vi "Test Cloneable API.vi"() -> ()   [LabVIEW 2024]
doc: "Cloneable API Tester."
uses:
  <vilib>/Utility/error.llb/DialogType.ctl
  <vilib>/JKI/JKI Simple Localization/Private/RegisterVIJKI_Simple_Localization.vi
  Cloneable.lvlib
  <vilib>/JKI/JKI Simple Localization/API/JKI Simple LocalizationJKI_Simple_Localization.lvlib
panel:
  out "last error":errorcluster
  in  "Show Diagram on Init":bool
  in  "wait for reply":bool=TRUE
  in  "Run as Singleton?":bool
  in  "Show Block Diagram":bool
  in  "Refresh Modules":bool
  in  "X":dbl=1.0
  out "Reply Payload":dbl
  out "Active Modules":string[](array[string])
  in  "Stop Module":bool
  in  "Select Module":i32(ring)=-1 caption="Select Module\nTo send Request to" items=["All"=-1, "1"=1, "2"=2, "3"=3, "4"=4, "5"=5, "6"=6, "7"=7, "8"=8, "9"=9, "10"=10]
  in  "Run New Module":bool
  out "Do Something Count":i32
  in  "Test Do Something Else and Wait for Reply":bool
  in  "Hide Module Panel":bool
  in  "Show Module Panel":bool caption="Show Panel"
  in  "Test Do Something Else":bool
  in  "Test Do Something":bool
  out "Status":string
  # "This VI tests the API for the Module."
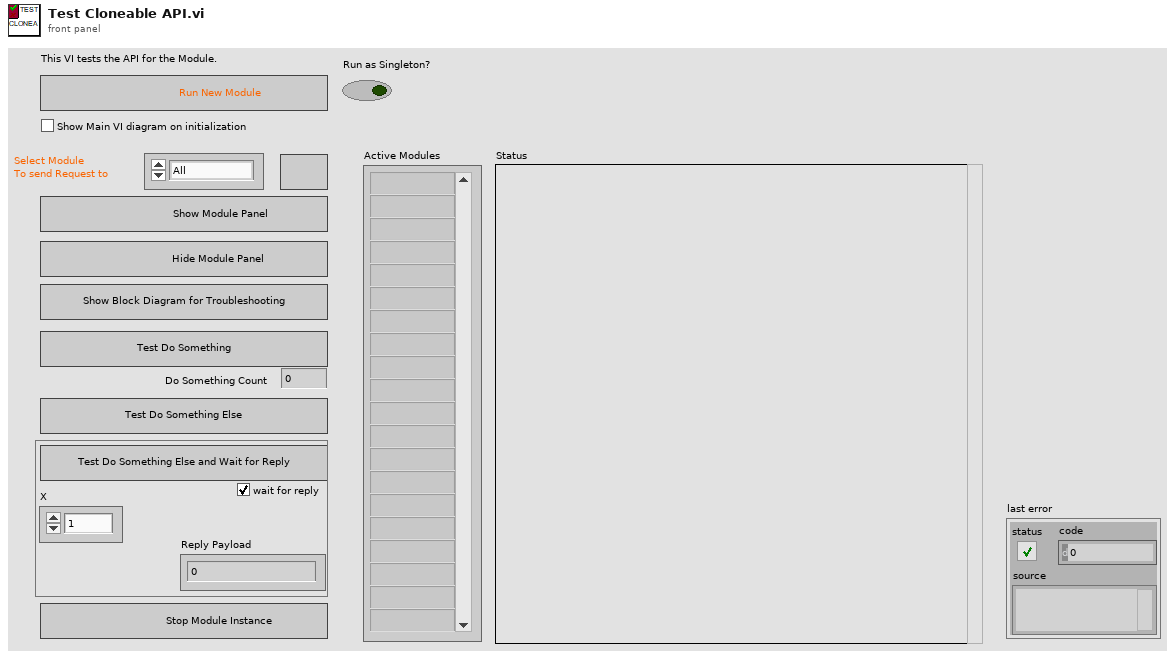
[diagram p1: front panel]
types:
  T1 = typedef "Cloneable.lvlib/Broadcast Events--cluster.ctl" = cluster{"Module Did Init":refnum<user-event>, "Status Updated":refnum<user-event>, "Error Reported":refnum<user-event>, "Did Something":refnum<user-event>, "Module Did Stop":refnum<user-event>, "Update Module Execution Status":refnum<user-event>}
  T2 = typedef "DialogType.ctl" = u16
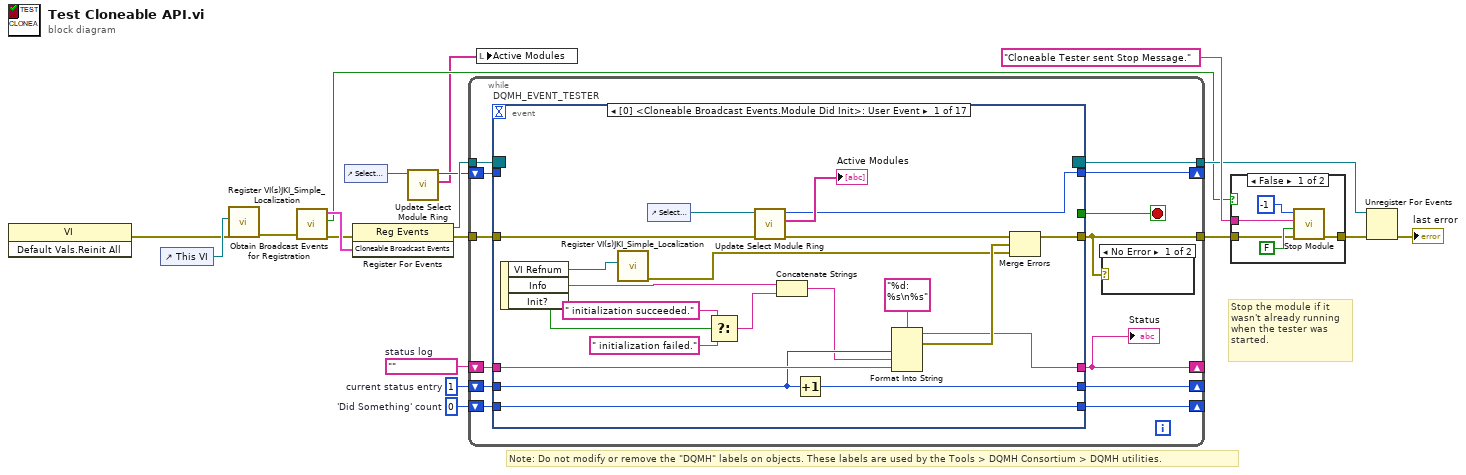
[diagram p0: block diagram]
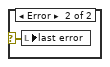
[diagram p3: hidden frame]
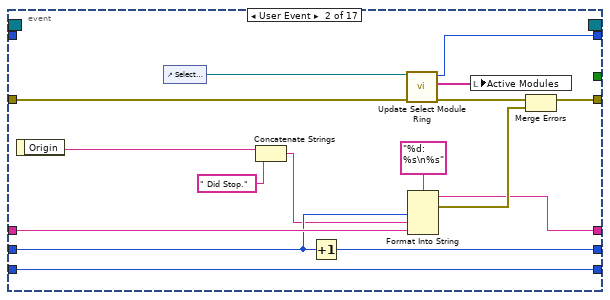
[diagram p4: hidden frame]
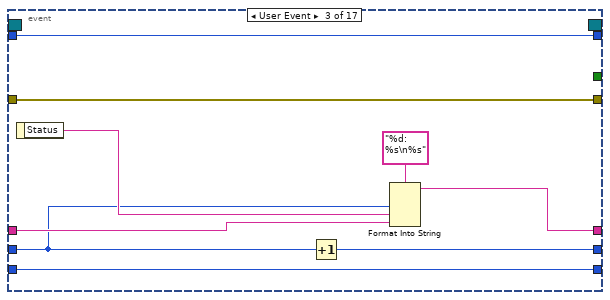
[diagram p5: hidden frame]
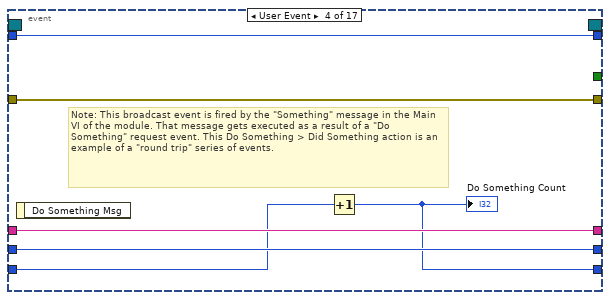
[diagram p6: hidden frame]
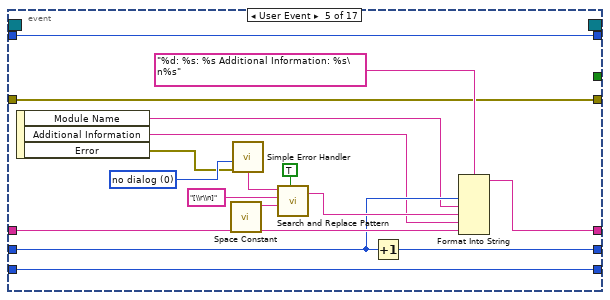
[diagram p7: hidden frame]
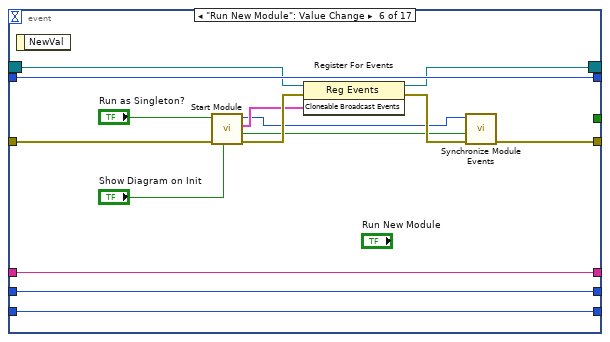
[diagram p8: hidden frame]
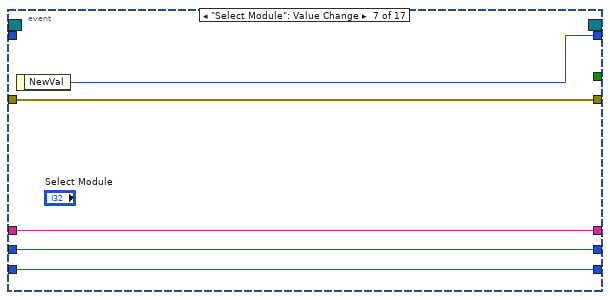
[diagram p9: hidden frame]
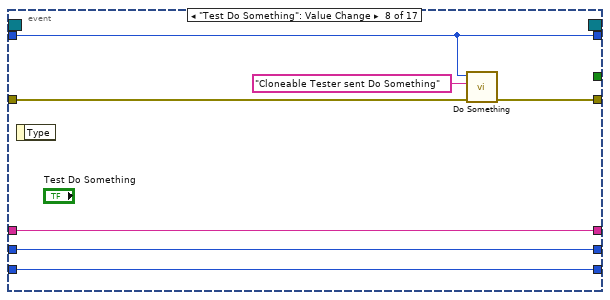
[diagram p10: hidden frame]
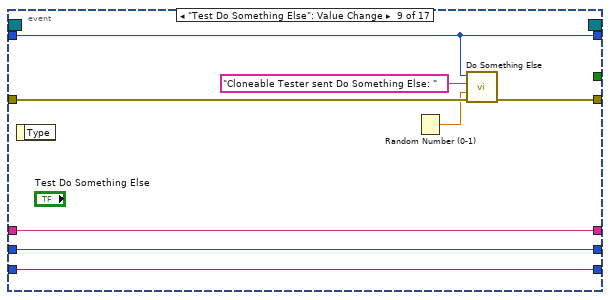
[diagram p11: hidden frame]
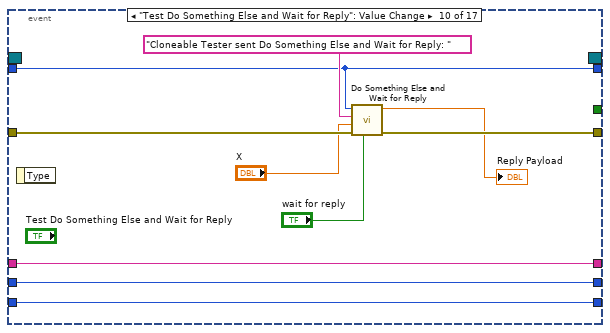
[diagram p12: hidden frame]
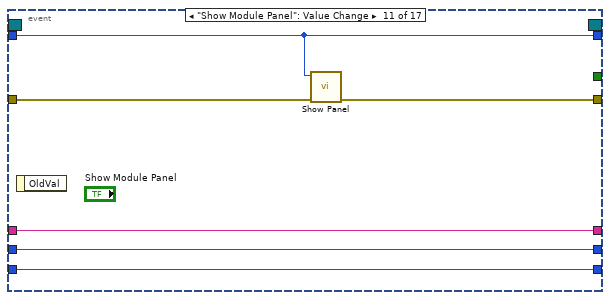
[diagram p13: hidden frame]
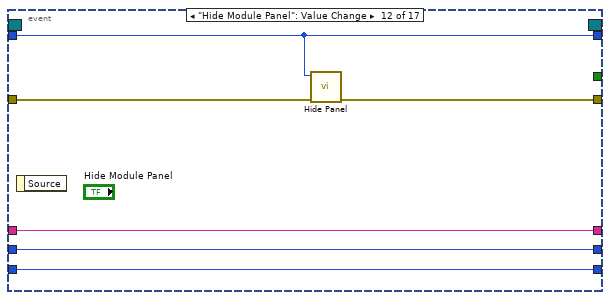
[diagram p14: hidden frame]
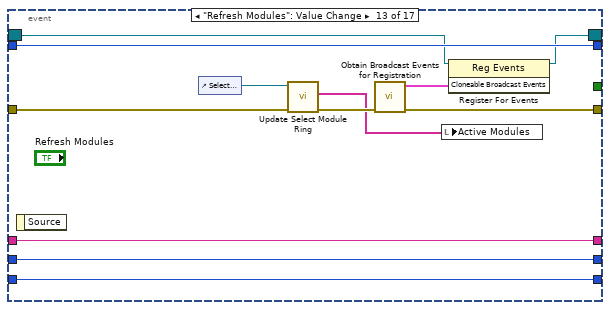
[diagram p15: hidden frame]
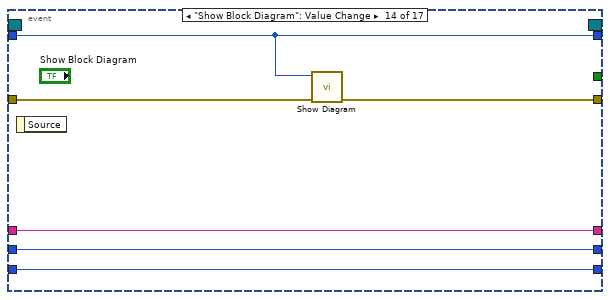
[diagram p16: hidden frame]
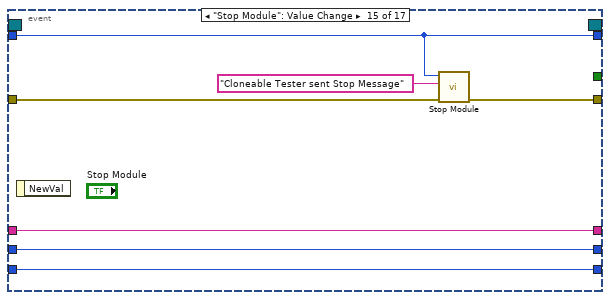
[diagram p17: hidden frame]
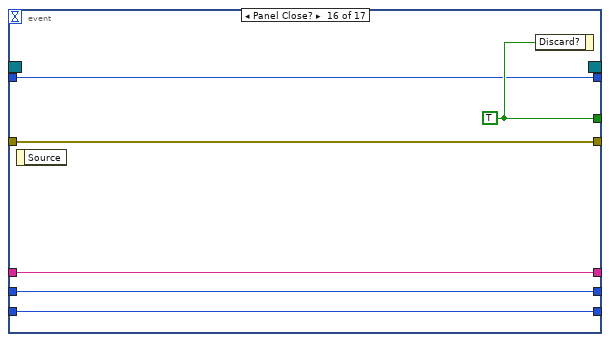
[diagram p18: hidden frame]
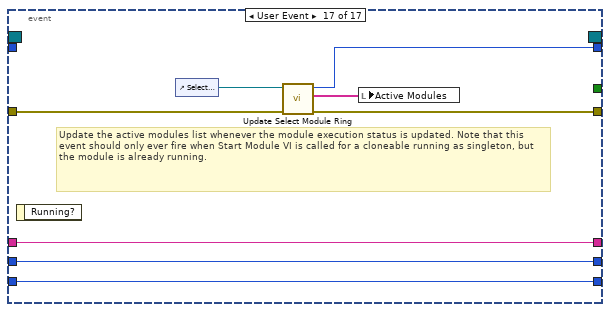
[diagram p19: hidden frame]
diagram:
  w15 = 0  # 'Did Something' count
  w16 = 1  # current status entry
  w17 = ""  # status log
  # "Stop the module if it wasn't already running when the tester was started."
  # "Note: Do not modify or remove the \"DQMH\" labels on objects. These labels are used by the Tools > DQMH Consortium > DQMH utilities."
  n1 = invoke class="VI" method="Default Vals.Reinit All"() -> (error out=w2:errorcluster)  [unwired: 3 in, 2 out]
  n2 = control-ref of="This VI"() -> (w3:refnum<vi>)
  n3 = call-poly <vilib>:"Register VI(s)JKI_Simple_Localization.vi"("error in"=w2, "VI Ref"=w3) -> ("error out"=w1:errorcluster)  [unwired: 8 in, 1 out]
  n4 = call "Obtain Broadcast Events for Registration.vi"("error in"=w1) -> ("error out"=w10:errorcluster, "Already running?"=w9:bool, "Cloneable Broadcast Events"=w14:T1)  [unwired: 8 in]
  n5 = control-ref of="Select Module"() -> (w6:refnum<vi>)
  n6 = register-events(error in=w10, w14) -> (reference out=w19:refnum<event-registration>, error out=w13:errorcluster)  [unwired: 1 in]
  n7 = call "Update Select Module Ring.vi"("Select Module Ring Ref"=w6) -> ("Active Modules (Array)"=w4:string[], "New Module Ring Value"=w5:i32)  [unwired: 8 in, 1 out]
  n8 = while {
    tunnel: w19 -> [w32]
    tunnel: [w21] -> w8
    tunnel: w13 -> [w31]
    shift-right: [w27] -> _
    shift-left: w17 -> [w29]
    shift-right: [w28] -> _
    shift-left: w16 -> [w30]
    shift-right: [w25] -> _
    shift-left: w15 -> [w26]
    shift-right: [w23] -> _
    shift-left: w5 -> [w24]
    tunnel: [w22] -> w11
    stop <- w20 stop-if-true
    n9 = event "DQMH_EVENT_TESTER" shown="[0] <Cloneable Broadcast Events.Module Did Init>: User Event" {
      selector: w32 -> [_ _ _ _ _ w110 _ _ _ _ _ _ w165 _ _ _ _]
      dyn-events: [_ _ _ _ _ w109 _ _ _ _ _ _ w164 _ _ _ _] -> w22
      timeout: _ -> [_ _ _ _ _ _ _ _ _ _ _ _ _ _ _ _ _]
      tunnel: [_ _ _ _ _ _ _ _ _ _ _ _ _ _ _ w190 _] -> w20
      tunnel: [w43 w61 w79 w85 w89 w108 w122 w128 w136 w147 w152 w158 w161 w173 w179 w189 w193] -> w21
      tunnel: w31 -> [w45 w63 w79 w85 w89 w111 w122 w129 w137 w141 w153 w159 w166 w177 w180 w189 w194]
      tunnel: w30 -> [w51 w67 w71 w83 w92 w114 w120 w125 w132 w144 w150 w156 w170 w175 w183 w187 w197]
      tunnel: w29 -> [w52 w68 w75 w84 w93 w115 w121 w126 w133 w145 w151 w157 w171 w176 w184 w188 w198]
      tunnel: [w49 w65 w76 w84 w91 w115 w121 w126 w133 w145 w151 w157 w171 w176 w184 w188 w198] -> w27
      tunnel: [w50 w66 w78 w83 w90 w114 w120 w125 w132 w144 w150 w156 w170 w175 w183 w187 w197] -> w28
      tunnel: w26 -> [w46 w64 w74 w82 w102 w113 w119 w124 w131 w143 w149 w155 w169 w174 w182 w186 w196]
      tunnel: [w46 w64 w74 w81 w102 w113 w119 w124 w131 w143 w149 w155 w169 w174 w182 w186 w196] -> w25
      tunnel: w24 -> [_ _ w72 w80 w101 w112 _ w123 w130 w142 w148 w154 w168 w172 w181 w185 _]
      tunnel: [w40 w58 w72 w80 w101 w112 w118 w123 w130 w142 w148 w154 w168 w172 w181 w185 w192] -> w23
      event User Event {
        n10 = event-data() -> ("VI Refnum"=w35:refnum<vi>, "Info"=w48:string, "Init?"=w37:bool)  [unwired: 1 in]
        n11 = call-poly <vilib>:"Register VI(s)JKI_Simple_Localization.vi"("VI Ref"=w35) -> ("error out"=w34:errorcluster)  [unwired: 9 in, 1 out]
        n12 = control-ref of="Select Module"() -> (w42:refnum<vi>)
        n13 = Select(t=" initialization succeeded.", s=w37, f=" initialization failed.") -> (s? t:f=w36:string)
        n14 = call "Update Select Module Ring.vi"("error in"=w45, "Select Module Ring Ref"=w42) -> ("error out"=w44:errorcluster, "Active Modules (Array)"=→"Active Modules":string[], "New Module Ring Value"=w40:i32)  [unwired: 7 in]
        n15 = Concatenate Strings(w48, w36) -> (w47:string)
        n16 = Increment(x=w51) -> (x+1=w50:i32)
        n17 = Format Into String(format string="%d: %s\n%s", w51, w47, w52) -> (resulting string=w49:string, error out=w54:errorcluster)  [unwired: 2 in]
        n18 = Merge Errors(w44, w54, w34) -> (w43:errorcluster)
      }
      event User Event {
        n19 = event-data() -> ("Origin"=w56:string)  [unwired: 1 in]
        n20 = control-ref of="Select Module"() -> (w60:refnum<vi>)
        n21 = Concatenate Strings(w56, " Did Stop.") -> (w55:string)
        n22 = Increment(x=w67) -> (x+1=w66:i32)
        n23 = call "Update Select Module Ring.vi"("error in"=w63, "Select Module Ring Ref"=w60) -> ("error out"=w62:errorcluster, "Active Modules (Array)"=w59:string[], "New Module Ring Value"=w58:i32)  [unwired: 7 in]
        n24 = Format Into String(format string="%d: %s\n%s", w67, w55, w68) -> (resulting string=w65:string, error out=w70:errorcluster)  [unwired: 2 in]
        n25 = local write "Active Modules"(w59) -> ()
        n26 = Merge Errors(w62, w70) -> (w61:errorcluster)
      }
      event User Event {
        n27 = event-data() -> ("Status"=w73:string)  [unwired: 1 in]
        n28 = Increment(x=w71) -> (x+1=w78:i32)
        n29 = Format Into String(format string="%d: %s\n%s", w71, w73, w75) -> (resulting string=w76:string)  [unwired: 2 in, 1 out]
      }
      event User Event {
        # "Note: This broadcast event is fired by the \"Something\" message in the Main VI of the module. That message gets executed as a result of a \"Do Something\" request event. This Do Something > Did Something action is an example of a \"round trip\" series of events."
        n30 = event-data() -> ()  [unwired: 1 in, 1 out]
        n31 = Increment(x=w82) -> (x+1=w81:i32)
        "Do Something Count" <- w81
      }
      event User Event {
        w94 = T2 0 items=["no dialog", "OK message", "continue or stop message", "OK message + warnings", "continue/stop + warnings"] ("type of dialog (OK msg:1)")
        n32 = event-data() -> ("Module Name"=w88:string, "Additional Information"=w87:string, "Error"=w86:errorcluster)  [unwired: 1 in]
        n33 = call <vilib>:"Space Constant.vi"() -> ("String"=w98:string)
        n34 = call <vilib>:"Simple Error Handler.vi"("type of dialog (OK msg:1)"=w94, "error in (no error)"=w86) -> ("message"=w95:string)  [unwired: 3 in, 4 out]
        n35 = call <vilib>:"Search and Replace Pattern.vi"("string"=w95, "regular expression (\"\")"="[\\r\\n]" ("regular expression (\"\")"), "replace string (\"\")"=w98, "replace all? (F)"=TRUE ("replace all CR/LF with spaces")) -> ("result string"=w96:string)  [unwired: 1 in, 1 out]
        n36 = Increment(x=w92) -> (x+1=w90:i32)
        n37 = Format Into String(format string="%d: %s: %s Additional Information: %s\n%s", w92, w88, w96, w87, w93) -> (resulting string=w91:string)  [unwired: 2 in, 1 out]
      }
      event "Run New Module": Value Change {
        n38 = event-data() -> ()  [unwired: 1 in, 1 out]
        n39 = call "Start Module.vi"("Show Main VI Diagram on Init (F)"="Show Diagram on Init", "error in"=w111, "Run as Singleton? (F)"="Run as Singleton?") -> ("error out"=w116:errorcluster, "Wait for Event Sync?"=w107:bool, "Cloneable Broadcast Events"=w106:T1, "Module ID"=w103:i32)  [unwired: 4 in, 1 out]
        n40 = register-events(reference=w110, error in=w116, w106) -> (reference out=w109:refnum<event-registration>, error out=w117:errorcluster)
        n41 = call "Synchronize Module Events.vi"("error in"=w117, "Wait for Event Sync?"=w107, "Module ID in"=w103) -> ("error out"=w108:errorcluster)  [unwired: 7 in, 1 out]
      }
      event "Select Module": Value Change {
        n42 = event-data() -> ("NewVal"=w118:i32)  [unwired: 1 in]
      }
      event "Test Do Something": Value Change {
        n43 = event-data() -> ()  [unwired: 1 in, 1 out]
        n44 = call "Do Something.vi"("error in"=w129, "Do Something Message"="Cloneable Tester sent Do Something", "Module ID"=w123) -> ("error out"=w128:errorcluster)  [unwired: 8 in]
      }
      event "Test Do Something Else": Value Change {
        n45 = event-data() -> ()  [unwired: 1 in, 1 out]
        n46 = Random Number (0-1)() -> (number: 0 to 1=w134:dbl)
        n47 = call "Do Something Else.vi"("error in"=w137, "X"=w134, "Do Something else Message"="Cloneable Tester sent Do Something Else: " ("Do Something Message"), "Module ID"=w130) -> ("error out"=w136:errorcluster)  [unwired: 7 in]
      }
      event "Test Do Something Else and Wait for Reply": Value Change {
        n48 = event-data() -> ()  [unwired: 1 in, 1 out]
        n49 = call "Do Something Else and Wait for Reply.vi"("wait for reply (T)"="wait for reply", "error in"=w141, "X"="X", "Do Something Else Message"="Cloneable Tester sent Do Something Else and Wait for Reply: " ("Do Something Message"), "Module ID"=w142) -> ("error out"=w147:errorcluster, "Value"=→"Reply Payload":dbl)  [unwired: 4 in, 1 out]
      }
      event "Show Module Panel": Value Change {
        n50 = event-data() -> ()  [unwired: 1 in, 1 out]
        n51 = call "Show Panel.vi"("error in"=w153, "Module ID"=w148) -> ("error out"=w152:errorcluster)  [unwired: 9 in]
      }
      event "Hide Module Panel": Value Change {
        n52 = event-data() -> ()  [unwired: 1 in, 1 out]
        n53 = call "Hide Panel.vi"("error in"=w159, "Module ID"=w154) -> ("error out"=w158:errorcluster)  [unwired: 9 in]
      }
      event "Refresh Modules": Value Change {
        n54 = event-data() -> ()  [unwired: 1 in, 1 out]
        n55 = control-ref of="Select Module"() -> (w167:refnum<vi>)
        n56 = call "Update Select Module Ring.vi"("error in"=w166, "Select Module Ring Ref"=w167) -> ("error out"=w162:errorcluster, "Active Modules (Array)"=w160:string[])  [unwired: 7 in, 1 out]
        n57 = call "Obtain Broadcast Events for Registration.vi"("error in"=w162) -> ("error out"=w161:errorcluster, "Cloneable Broadcast Events"=w163:T1)  [unwired: 8 in, 1 out]
        n58 = local write "Active Modules"(w160) -> ()
        n59 = register-events(reference=w165, w163) -> (reference out=w164:refnum<event-registration>)  [unwired: 1 in, 1 out]
      }
      event "Show Block Diagram": Value Change {
        n60 = event-data() -> ()  [unwired: 1 in, 1 out]
        n61 = call "Show Diagram.vi"("error in"=w177, "Module ID"=w172) -> ("error out"=w173:errorcluster)  [unwired: 9 in]
      }
      event "Stop Module": Value Change {
        n62 = event-data() -> ()  [unwired: 1 in, 1 out]
        n63 = call "Stop Module.vi"("error in"=w180, "Origin"="Cloneable Tester sent Stop Message", "Module ID"=w181) -> ("error out"=w179:errorcluster)  [unwired: 8 in]
      }
      event Panel Close? {
        w190 = TRUE ("Discard?")
        n64 = event-data() -> ()  [unwired: 1 in, 1 out]
        n65 = event-data("Discard?"=w190) -> ()  [unwired: 1 in, 1 out]
      }
      event User Event {
        # "Update the active modules list whenever the module execution status is updated. Note that this event should only ever fire when Start Module VI is called for a cloneable running as singleton, but the module is already running."
        n66 = event-data() -> ()  [unwired: 1 in, 1 out]
        n67 = control-ref of="Select Module"() -> (w195:refnum<vi>)
        n68 = call "Update Select Module Ring.vi"("error in"=w194, "Select Module Ring Ref"=w195) -> ("error out"=w193:errorcluster, "Active Modules (Array)"=w191:string[], "New Module Ring Value"=w192:i32)  [unwired: 7 in]
        n69 = local write "Active Modules"(w191) -> ()
      }
    }
    "Status" <- w27
    n70 = case shown="No Error" w21 {
      selector: w21 -> [_ w33]
      frame No Error {
      }
      frame Error {
        n71 = local write "last error"(w33) -> ()
      }
    }
  }
  n72 = local write "Active Modules"(w4) -> ()
  n73 = case shown="False" w9 {
    tunnel: [w203 w204] -> w18
    tunnel: "Cloneable Tester sent Stop Message." ("Origin") -> [w202 _]
    tunnel: w8 -> [w199 w204]
    frame False {
      n74 = call "Stop Module.vi"("error in"=w199, "Wait for Module to stop? (F)"=FALSE ("Wait for Module to stop?"), "Origin"=w202, "Module ID"=-1 ("Stop all")) -> ("error out"=w203:errorcluster)  [unwired: 7 in]
    }
    frame True {
    }
  }
  n75 = Unregister For Events(event registration refnum=w11, error in=w18) -> (error out=→"last error":errorcluster)
